vi "Send Command.vi"(8 "error in":errorcluster, 9 "Disable register writing (T)":bool=TRUE, 10 "Command":string, 11 "VISA Session In":refnum<visa-resource-name>="Alicat") -> (0 "error out":errorcluster, 2 "Response":string, 3 "VISA Session Out":refnum<visa-resource-name>)   [LabVIEW 2016]
doc: "Sends the specified text command to an Alicat device. Register writes are disabled by default, but can be enabled by wiring a false constant to the \"Disable register writing\" terminal. Returns Alicat response as a string (unedited)."
uses:
  <vilib>/Instr/_visa.llb/VISA Flush IO Buffer Mask.ctl
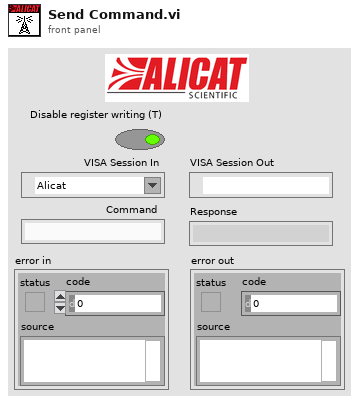
[diagram p1: front panel]
types:
  T1 = typedef "VISA Flush IO Buffer Mask.ctl" = u16
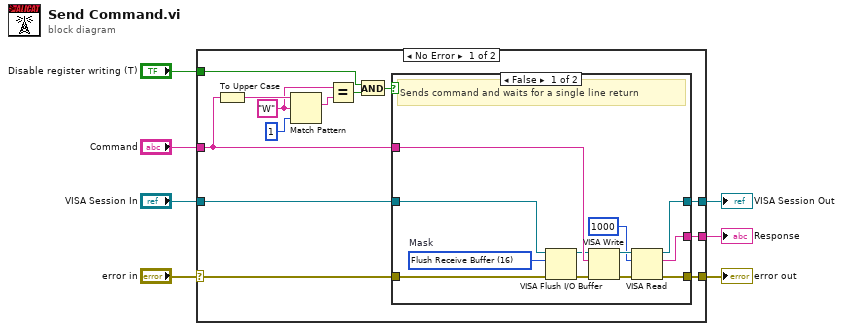
[diagram p0: block diagram]
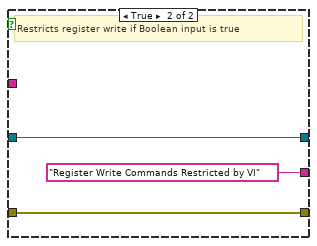
[diagram p2: hidden frame]
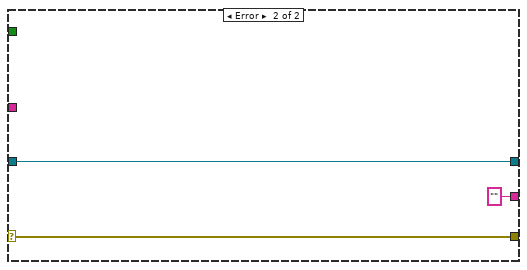
[diagram p3: hidden frame]
diagram:
  n1 = case shown="No Error" "error in" {
    selector: "error in" -> [w10 w37]
    tunnel: [w20 w37] -> w7
    tunnel: [w19 "" ("read buffer")] -> w6
    tunnel: "Command" -> [w16 _]
    tunnel: "Disable register writing (T)" -> [w11 _]
    tunnel: [w9 w36] -> w2
    tunnel: "VISA Session In" -> [w8 w36]
    frame No Error {
      w15 = "W" ("regular expression")
      n2 = To Upper Case(1:w16) -> (0:w17:string)
      n3 = Match Pattern(string=w17, regular expression=w15, offset (0)=1) -> (match substring=w14:string)  [unwired: 3 out]
      n4 = Equal?(x=w15, y=w14) -> (x = y?=w13:bool)
      n5 = And(x=w11, y=w13) -> (x .and. y?=w12:bool)
      n6 = case shown="False" w12 {
        tunnel: w10 -> [w32 w34]
        tunnel: [w31 w34] -> w20
        tunnel: [w30 "Register Write Commands Restricted by VI" ("read buffer")] -> w19
        tunnel: w16 -> [w29 _]
        tunnel: [w22 w33] -> w9
        tunnel: w8 -> [w21 w33]
        frame False {
          w23 = T1 16 items=["Flush Receive Buffer"=16, "Write Transmit Buffer to Device"=32, "Flush Receive Buffer (No I/O)"=64, "Flush Transmit Buffer"=128]  # Mask
          # "Sends command and waits for a single line return"
          n7 = VISA Flush I/O Buffer(VISA resource name=w21, mask (16)=w23, error in (no error)=w32) -> (VISA resource name out=w27:refnum<visa-resource-name>, error out=w24:errorcluster)
          n8 = VISA Write(VISA resource name=w27, write buffer=w29, error in (no error)=w24) -> (VISA resource name out=w26:refnum<visa-resource-name>, error out=w28:errorcluster)  [unwired: 1 out]
          n9 = VISA Read(VISA resource name=w26, byte count=u32 1000, error in (no error)=w28) -> (VISA resource name out=w22:refnum<visa-resource-name>, read buffer=w30:string, error out=w31:errorcluster)  [unwired: 1 out]
        }
        frame True {
          # "Restricts register write if Boolean input is true"
        }
      }
    }
    frame Error {
    }
  }
  "error out" <- w7
  "Response" <- w6
  "VISA Session Out" <- w2
